vi "ExtractData.vi"(8 "Samples per freq calc":i32=10000, 9 "Samples to average":i32, 11 "Data input":waveform(dbl)[](array[waveform])) -> (3 "Data cluster":T1)   [LabVIEW 2019]
uses:
  <vilib>/measure/madcrms.llb/Basic Averaged DC-RMS for 1 Chan.vi
  <vilib>/gmath/NI_Gmath.lvlib
  <vilib>/measure/NI_MAPro.lvlib
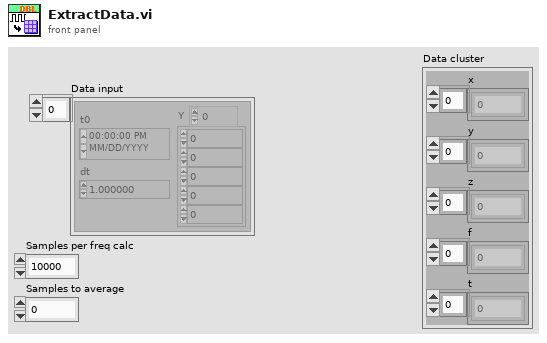
[diagram p1: front panel]
types:
  T1 = cluster{"x":dbl[], "y":dbl[], "z":dbl[], "f":dbl[], "t":dbl[]}
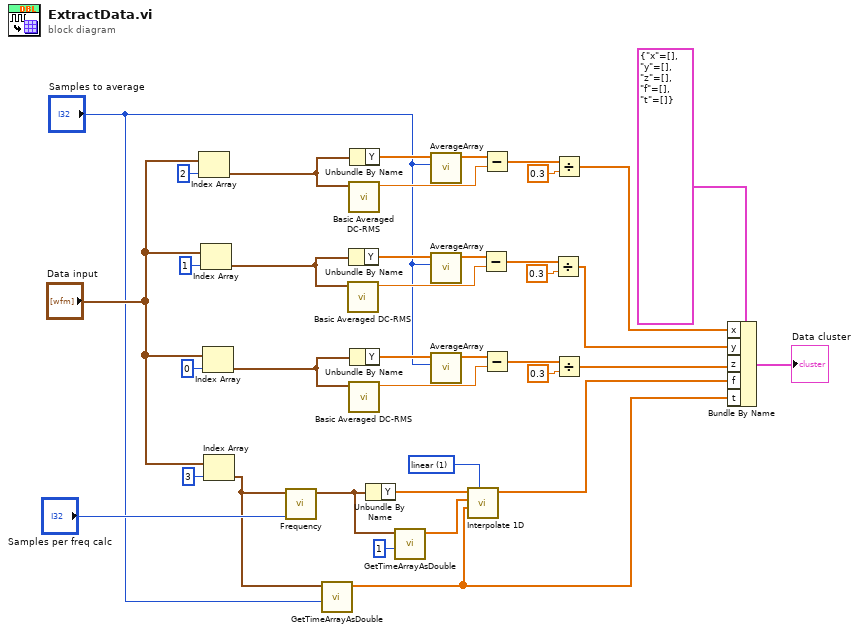
[diagram p0: block diagram]
diagram:
  w36 = 1 items=["nearest", "linear", "spline", "cubic Hermite", "Lagrange"] ("method")
  n1 = Index Array(array="Data input", index=2) -> (element=w15:waveform(dbl))
  n2 = Index Array(array="Data input", index=1) -> (element=w16:waveform(dbl))
  n3 = Index Array(array="Data input", index=0) -> (element=w17:waveform(dbl))
  n4 = Index Array(array="Data input", index=3) -> (element=w14:waveform(dbl))
  n5 = call "Frequency.vi"("Samples per calculation"="Samples per freq calc", "Input waveform"=w14) -> ("Frequency waveform"=w37:waveform(dbl))  [unwired: 9 in]
  n6 = call "GetTimeArrayAsDouble.vi"("Get every n-th"="Samples to average", "Waveform"=w14) -> ("Time Array"=w3:dbl[])  [unwired: 9 in]
  n7 = call-poly <vilib>:"Basic Averaged DC-RMS.vi"("signal in"=w16) -> ("DC value"=w28:dbl)  [unwired: 7 in, 3 out]
  n8 = call-poly <vilib>:"Basic Averaged DC-RMS.vi"("signal in"=w15) -> ("DC value"=w32:dbl)  [unwired: 7 in, 3 out]
  n9 = Unbundle By Name(w16) -> ("Y"=w29:dbl[])
  n10 = call-poly <vilib>:"Basic Averaged DC-RMS.vi"("signal in"=w17) -> ("DC value"=w24:dbl)  [unwired: 7 in, 3 out]
  n11 = Unbundle By Name(w15) -> ("Y"=w33:dbl[])
  n12 = Unbundle By Name(w17) -> ("Y"=w25:dbl[])
  n13 = Unbundle By Name(w37) -> ("Y"=w8:dbl[])
  n14 = call "GetTimeArrayAsDouble.vi"("Get every n-th"=1, "Waveform"=w37) -> ("Time Array"=w38:dbl[])  [unwired: 9 in]
  n15 = call "AverageArray.vi"("Samples to average"="Samples to average", "Data in"=w33) -> ("Data out"=w13:dbl[])  [unwired: 9 in]
  n16 = call "AverageArray.vi"("Samples to average"="Samples to average", "Data in"=w29) -> ("Data out"=w12:dbl[])  [unwired: 9 in]
  n17 = call "AverageArray.vi"("Samples to average"="Samples to average", "Data in"=w25) -> ("Data out"=w11:dbl[])  [unwired: 9 in]
  n18 = call <vilib>:"Interpolate 1D.vi"("method"=w36, "xi"=w3, "X"=w38, "Y"=w8) -> ("yi"=w4:dbl[])  [unwired: 5 in, 2 out]
  n19 = Subtract(x=w12, y=w28) -> (x-y=w30:dbl[])
  n20 = Subtract(x=w13, y=w32) -> (x-y=w34:dbl[])
  n21 = Subtract(x=w11, y=w24) -> (x-y=w26:dbl[])
  n22 = Divide(x=w30, y=0.3) -> (x/y=w6:dbl[])
  n23 = Divide(x=w34, y=0.3) -> (x/y=w7:dbl[])
  n24 = Divide(x=w26, y=0.3) -> (x/y=w5:dbl[])
  n25 = Bundle By Name(cluster=T1 {"x"=[], "y"=[], "z"=[], "f"=[], "t"=[]} ("input cluster"), "x"=w7, "y"=w6, "z"=w5, "f"=w4, "t"=w3) -> (→"Data cluster":T1)
